vi "Fit_1D_Gaussian.vi"(0 "Input 1D Array":dbl[](array[numeric])) -> (2 "center":dbl, 3 "FWHM":dbl format="%#.1g")   [LabVIEW 2015]
panel:
  out "RMS":dbl
  out "Gaussian Fit":dbl[](array[numeric])
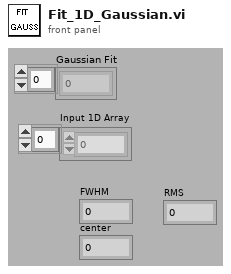
[diagram p1: front panel]
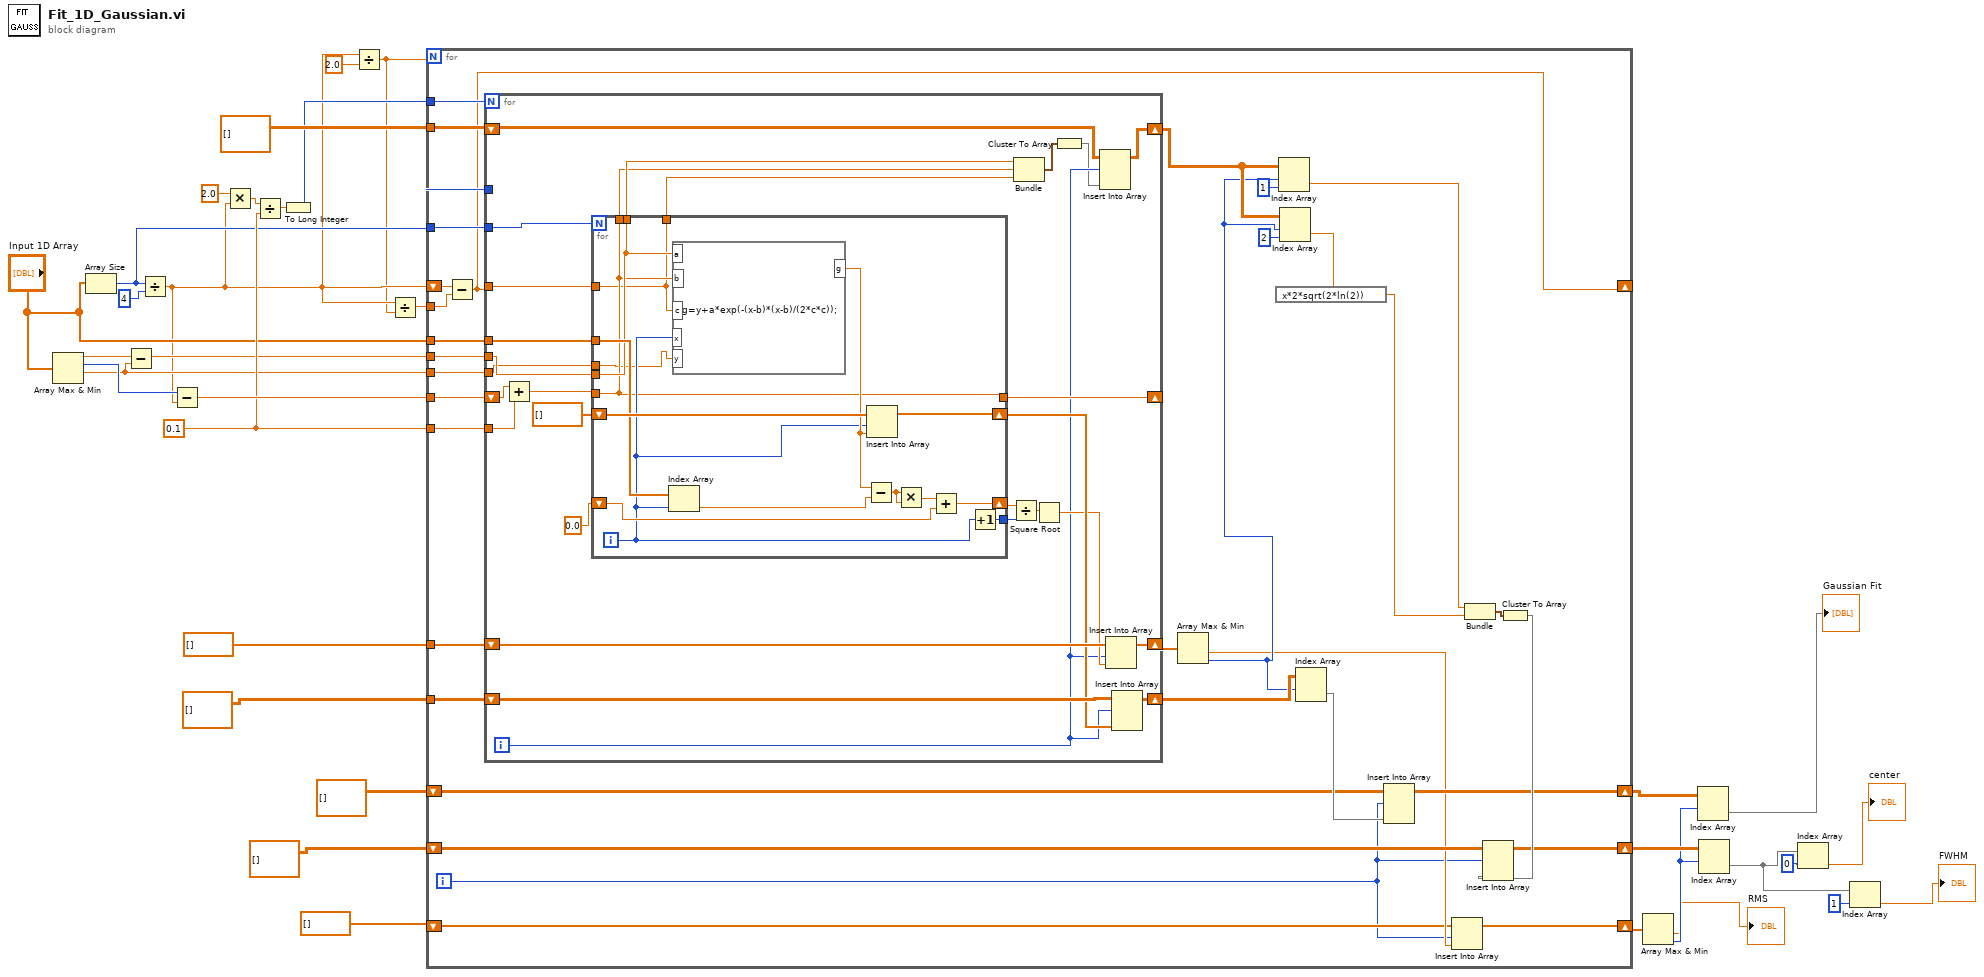
[diagram p0: block diagram]
diagram:
  w29 = 0.1 ("y")
  n1 = Array Max & Min(array="Input 1D Array") -> (max value=w24:dbl, max index (indices)=w33:i32, min value=w23:dbl)  [unwired: 1 out]
  n2 = Array Size(array="Input 1D Array") -> (size(s)=w20:i32)
  n3 = Subtract(x=w24, y=w23) -> (x-y=w22:dbl)
  n4 = Divide(x=w20, y=4) -> (x/y=w3:dbl)
  n5 = Subtract(x=w33, y=w3) -> (x-y=w32:dbl)
  n6 = Multiply(x=2.0, y=w3) -> (x*y=w30:dbl)
  n7 = Divide(x=w30, y=w29) -> (x/y=w28:dbl)
  n8 = To Long Integer(number=w28) -> (32bit integer=w21:i32)
  n9 = Divide(x=w3, y=2.0) -> (x/y=w2:dbl)
  n10 = Divide(x=w3, y=w2) -> (x/y=w1:dbl)
  n11 = for {
    N: w2 -> [_]
    tunnel: "Input 1D Array" -> [w67]
    tunnel: w32 -> [w66]
    tunnel: w29 -> [w65]
    tunnel: dbl[] [] -> [w64]
    tunnel: dbl[][] [] -> [w62]
    tunnel: dbl[][] [] -> [w60]
    tunnel: w23 -> [w54]
    tunnel: w22 -> [w53]
    tunnel: w21 -> [w52]
    tunnel: w20 -> [w51]
    shift-right: [w49] -> _
    shift-left: w3 -> [w50]
    shift-right: [w42] -> w15
    shift-left: dbl[][] [] -> [w48]
    shift-right: [w41] -> w16
    shift-left: dbl[][] [] -> [w40]
    shift-right: [w37] -> w14
    shift-left: dbl[] [] -> [w38]
    tunnel: w1 -> [w35]
    i -> [w36]
    n12 = Subtract(x=w50, y=w35) -> (x-y=w49:dbl)
    n13 = for {
      N: w52 -> [_]
      tunnel: w53 -> [w95]
      tunnel: w67 -> [w94]
      tunnel: w49 -> [w88]
      tunnel: w65 -> [w85]
      shift-right: [w84] -> _
      shift-left: w66 -> [w86]
      shift-right: [w79] -> w63
      shift-left: w64 -> [w80]
      shift-right: [w76] -> w61
      shift-left: w62 -> [w78]
      shift-right: [w73] -> w57
      shift-left: w60 -> [w72]
      tunnel: w54 -> [w71]
      tunnel: w52 -> [_]
      tunnel: w51 -> [w70]
      i -> [w74]
      n14 = Add(x=w86, y=w85) -> (x+y=w87:dbl)
      n15 = for {
        N: w70 -> [_]
        tunnel: w94 -> [w108]
        tunnel: w95 -> [w99]
        tunnel: w87 -> [w98]
        shift-right: [w109] -> w77
        shift-left: dbl[] [] -> [w110]
        tunnel: w88 -> [w97]
        shift-right: [w102] -> w91
        shift-left: 0.0 ("y") -> [w103]
        tunnel: [w100] -> w90
        tunnel: [w98] -> w84
        tunnel: [w99] -> w83
        tunnel: [w98] -> w82
        tunnel: [w97] -> w81
        tunnel: w71 -> [w96]
        i -> [w101]
        n16 = Index Array(array=w108, index=w101) -> (element=w106:dbl)
        n17 = formula code="g=y+a*exp(-(x-b)*(x-b)/(2*c*c));"("a"=w99, "b"=w98, "c"=w97, "x"=w101, "y"=w96) -> ("g"=w107:dbl)
        n18 = Subtract(x=w107, y=w106) -> (x-y=w105:dbl)
        n19 = Insert Into Array(array=w110, index=w101, new element=w107) -> (w109:dbl[])
        n20 = Multiply(x=w105, y=w105) -> (x*y=w104:dbl)
        n21 = Add(x=w104, y=w103) -> (x+y=w102:dbl)
        n22 = Increment(x=w101) -> (x+1=w100:i32)
      }
      n23 = Divide(x=w91, y=w90) -> (x/y=w89:dbl)
      n24 = Bundle(w83, w82, w81) -> (w69:cluster{dbl, dbl, dbl})  [unwired: 1 in]
      n25 = Square Root(x=w89) -> (sqrt(x)=w75:dbl)
      n26 = Cluster To Array(cluster=w69) -> (array=w68:dbl[])
      n27 = Insert Into Array(array=w72, index (row)=w74, new element=w68) -> (w73:dbl[][])  [unwired: 1 in]
      n28 = Insert Into Array(array=w80, index=w74, new element=w75) -> (w79:dbl[])
      n29 = Insert Into Array(array=w78, index (row)=w74, new element=w77) -> (w76:dbl[][])  [unwired: 1 in]
    }
    n30 = Array Max & Min(array=w63) -> (min value=w39:dbl, min index (indices)=w55:i32)  [unwired: 2 out]
    n31 = Index Array(array=w57, index (row)=w55, index (col)=1 ("disabled index (col)")) -> (element=w45:dbl)
    n32 = Index Array(array=w57, index (row)=w55, index (col)=2 ("disabled index (col)")) -> (element=w56:dbl)
    n33 = expression code="x*2*sqrt(2*ln(2))"(w56) -> (w44:dbl)
    n34 = Index Array(array=w61, index (row)=w55) -> (element=w47:dbl[])  [unwired: 1 in]
    n35 = Insert Into Array(array=w40, index (row)=w36, new element=w47) -> (w41:dbl[][])  [unwired: 1 in]
    n36 = Insert Into Array(array=w38, index=w36, new element=w39) -> (w37:dbl[])
    n37 = Bundle("g"=w45, "g"=w44) -> (w46:cluster{"g":dbl, "g":dbl})  [unwired: 1 in]
    n38 = Cluster To Array(cluster=w46) -> (array=w43:dbl[])
    n39 = Insert Into Array(array=w48, index (row)=w36, new element=w43) -> (w42:dbl[][])  [unwired: 1 in]
  }
  n40 = Array Max & Min(array=w14) -> (min value=→"RMS":dbl, min index (indices)=w13:i32)  [unwired: 2 out]
  n41 = Index Array(array=w16, index (row)=w13) -> (element=→"Gaussian Fit":dbl[])  [unwired: 1 in]
  n42 = Index Array(array=w15, index (row)=w13) -> (element=w7:dbl[])  [unwired: 1 in]
  n43 = Index Array(array=w7, index=0 ("index (row)")) -> (element=→"center":dbl)
  n44 = Index Array(array=w7, index=1 ("index (row)")) -> (element=→"FWHM":dbl)
